vi "Get Environment.vi"(8 "error in":errorcluster, 10 "?":T1, 11 "Paths":T2) -> (0 "error out":errorcluster, 3 "Environment out":refnum<k24>)   [LabVIEW 2020, in "WebView2.lvlib" / "WebView2 Control.lvclass"]
uses:
  WebView2 Control.lvclass
  C:/Users/Simon/Documents/GitHub/LV-WebView2/Source/Libs/Microsoft.Web.WebView2.Core.dll
  Libs/Microsoft.Web.WebView2.Core.dll
  <vilib>/ErrorRing/Error Ring.xnode
  WebView2 Control.lvclass/WebView2 Control.ctl
  <vilib>/Utility/error.llb/Error Cluster From Error Code.vi
  Paths.ctl
  Core Env Options.ctl
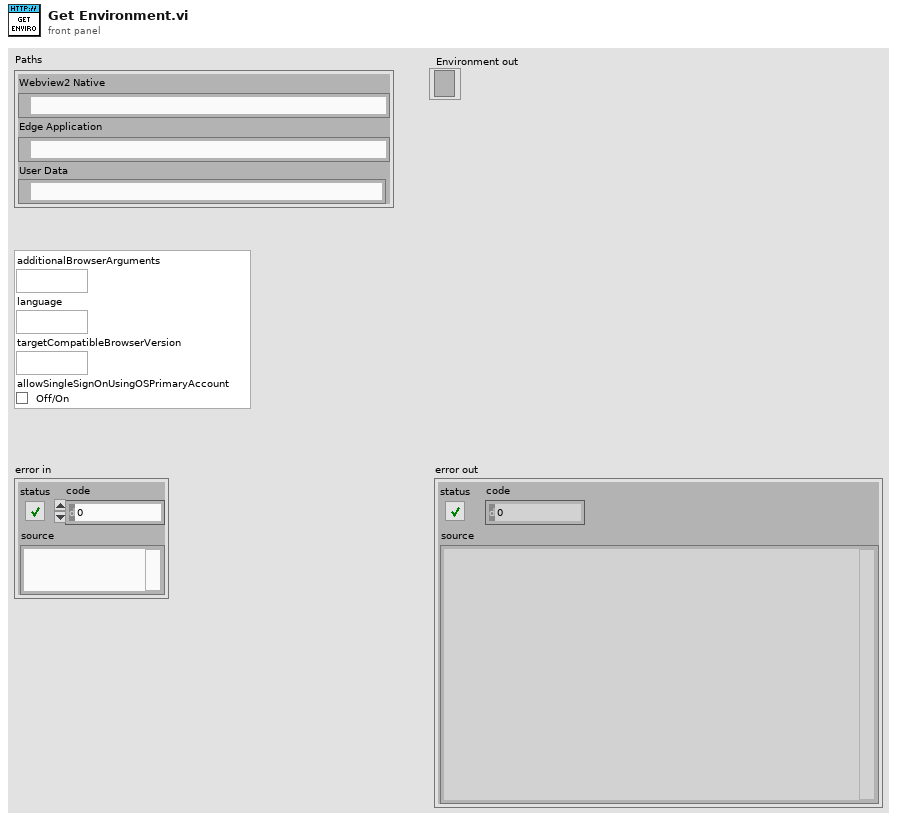
[diagram p1: front panel]
types:
  T1 = typedef "WebView2.lvlib/WebView2 Control.lvclass/Core Env Options.ctl" = cluster{"additionalBrowserArguments":string, "language":string, "targetCompatibleBrowserVersion":string, "allowSingleSignOnUsingOSPrimaryAccount":bool}
  T2 = typedef "WebView2.lvlib/WebView2 Control.lvclass/Paths.ctl" = cluster{"Webview2 Native":path, "Edge Application":path, "User Data":path}
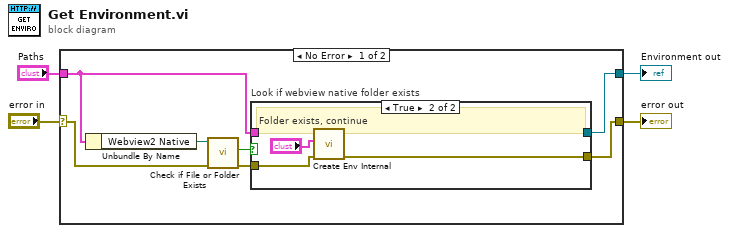
[diagram p0: block diagram]
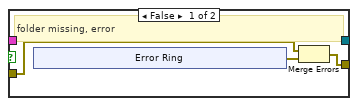
[diagram p2: hidden frame]
diagram:
  n1 = case shown="No Error" "error in" {
    selector: "error in" -> [w8 w24]
    tunnel: [w11 w24] -> w4
    tunnel: [w10 _] -> w3
    tunnel: "Paths" -> [w9 _]
    frame No Error {
      n2 = Unbundle By Name(w9) -> ("Webview2 Native"=w6:path)
      n3 = call <vilib>:"Check if File or Folder Exists.vi"("error in (no error)"=w8, "path"=w6) -> ("error out"=w7:errorcluster, "file or folder exists?"=w5:bool)  [unwired: 7 in, 1 out]
      n4 = case "Look if webview native folder exists" shown="True" w5 {
        tunnel: w7 -> [w14 w23]
        tunnel: [w13 w21] -> w11
        tunnel: [_ w19] -> w10
        tunnel: w9 -> [_ w20]
        frame False {
          # "folder missing, error"
          n5 = xnode "Error Ring"() -> ("error out"=w12:errorcluster)
          n6 = Merge Errors(w14, w12) -> (w13:errorcluster)
        }
        frame True {
          # "Folder exists, continue"
          n7 = call "Create Env Internal.vi"("error in (no error)"=w23, 10:"?", "Paths"=w20) -> ("error out"=w21:errorcluster, "Env"=w19:refnum<k24>)  [unwired: 7 in]
        }
      }
    }
    frame Error {
    }
  }
  "error out" <- w4
  "Environment out" <- w3
